vi "AVI Video Close.vi"(8 "error in (no error)":errorcluster, 11 "Channel":T1) -> (0 "error out":errorcluster)   [LabVIEW 2013]
uses:
  Typedefs/Channel Selector.ctl
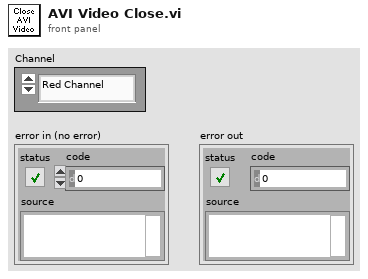
[diagram p1: front panel]
types:
  T1 = typedef "Channel Selector.ctl" = enum16{"Red Channel", "Green Channel", "Blended"}
  T2 = typedef "AVI implementation enum.ctl" = enum16{"AVI1", "AVI2"}
  T3 = typedef "AVI Refs cluster.ctl" = cluster{"AVI2 path":path, "AVI 2 Refnum":T4, "New Image":T5, "error out":errorcluster, "Avi 1 Refnum":T6}
  T4 = typedef "IMAQ AVI2 Refnum.ctl" = refnum<k20>
  T5 = typedef "IMAQ Image.ctl" = refnum<image>
  T6 = typedef "AviRefnum.ctl" = refnum<k1>
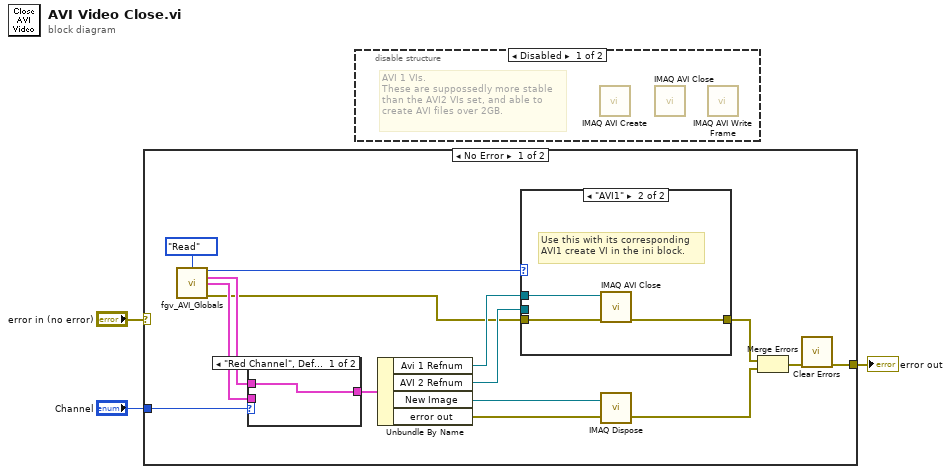
[diagram p0: block diagram]
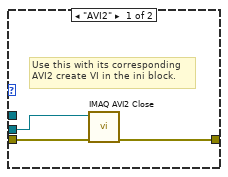
[diagram p2: hidden frame]
diagram:
  n1 = case shown="No Error" "error in (no error)" {
    selector: "error in (no error)" -> [_ w27]
    tunnel: "Channel" -> [w4 _]
    tunnel: [w5 w27] -> w1
    frame No Error {
      n2 = call "fgv_AVI_Globals.vi"("Function"=enum16{"Intialize", "Write", "Read", "Clear"}."Read") -> ("AVI mode"=w14:T2, "Red AVI"=w16:T3, "Green AVI"=w15:T3, "error out"=w6:errorcluster)  [unwired: 11 in]
      n3 = case shown="\"Red Channel\", Default" w4 {
        tunnel: [w25 w26] -> w18
        tunnel: w16 -> [w25 _]
        tunnel: w15 -> [_ w26]
        frame "Red Channel", Default {
        }
        frame "Green Channel" {
        }
      }
      n4 = Unbundle By Name(w18) -> ("Avi 1 Refnum"=w8:T6, "AVI 2 Refnum"=w12:T4, "New Image"=w11:T5, "error out"=w13:errorcluster)
      n5 = case shown="\"AVI2\"" w14 {
        tunnel: w12 -> [w21 _]
        tunnel: [w20 w24] -> w9
        tunnel: w6 -> [w19 w23]
        tunnel: w8 -> [_ w22]
        frame "AVI2" {
          # "Use this with its corresponding\nAVI2 create VI in the ini block."
          n6 = call "IMAQ AVI2 Close"("error in (no error)"=w19, "AVI Refnum"=w21) -> ("error out"=w20:errorcluster)  [unwired: 9 in]
        }
        frame "AVI1" {
          # "Use this with its corresponding\nAVI1 create VI in the ini block."
          n7 = call "IMAQ AVI Close"("error in (no error)"=w23, "Avi Refnum"=w22) -> ("error out"=w24:errorcluster)  [unwired: 9 in]
        }
      }
      n8 = call "IMAQ Dispose"("Image"=w11, "error in (no error)"=w13) -> ("error out"=w10:errorcluster)  [unwired: 4 in]
      n9 = Merge Errors(w9, w10) -> (w7:errorcluster)
      n10 = call <vilib>:"Clear Errors.vi"("error in (no error)"=w7) -> ("error out"=w5:errorcluster)  [unwired: 6 in]
    }
    frame Error {
    }
  }
  "error out" <- w1
  n11 = disable-structure shown="Disabled" {
    frame Disabled {
      # "AVI 1 VIs.\nThese are suppossedly more stable\nthan the AVI2 VIs set, and able to\ncreate AVI files over 2GB."
      n12 = call "IMAQ AVI Create"() -> ()  [unwired: 10 in, 2 out]
      n13 = call "IMAQ AVI Close"() -> ()  [unwired: 11 in, 1 out]
      n14 = call "IMAQ AVI Write Frame"() -> ()  [unwired: 10 in, 2 out]
    }
    frame Enabled {
    }
  }
